vi "saturatearray.vi"(0 "S1in in":u16=15000 min=10240 max=19650 step=100, 5 "S2in in":u16=15000 min=10240 max=19650 step=100, 7 "S3in in":u16=15000 min=10240 max=19650 step=100, 9 "S4in in":u16=15000 min=10240 max=19650 step=100, 11 "S5in in":u16=15000 min=10240 max=19650 step=100) -> (4 "S1in out":u16, 6 "S2in out":u16, 8 "S3in out":u16, 10 "S4in out":u16, 15 "S5in out":u16)   [LabVIEW 2011]
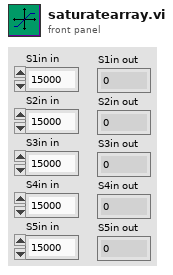
[diagram p1: front panel]
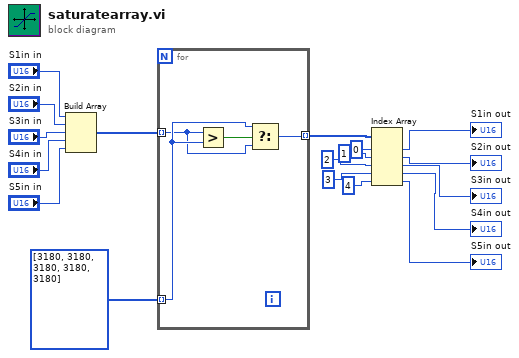
[diagram p0: block diagram]
diagram:
  n1 = Build Array("S1in in", "S2in in", "S3in in", "S4in in", "S5in in") -> (w12:u16[])
  n2 = for {
    tunnel: i32[] [3180, 3180, 3180, 3180, 3180] -> [w21] mode=indexing
    tunnel: w12 -> [w20] mode=indexing
    tunnel: [w19] -> w1 mode=indexing
    n3 = Greater?(x=w20, y=w21) -> (0:w22:bool)
    n4 = Select(t=w21, s=w22, f=w20) -> (s? t:f=w19:i32)
  }
  n5 = Index Array(array=w1, index #1=0 ("index"), index #2=1 ("index"), index #3=2 ("index"), index #4=3 ("index"), index #5=4 ("index")) -> (element #1=→"S1in out":i32, element #2=→"S2in out":i32, element #3=→"S3in out":i32, element #4=→"S4in out":i32, element #5=→"S5in out":i32)
